vi "Close.vi"(8 "error in (no error)":errorcluster, 11 "HTS221 in":refnum<class "HTS221.lvclass">) -> (0 "error out":errorcluster, 3 "HTS221 out":refnum<class "HTS221.lvclass">)   [LabVIEW 2020, in "HTS221.lvclass"]
doc: "Disables the HTS221"
uses:
  HTS221.lvclass
  LINX I2C/LINX I2C.lvclass
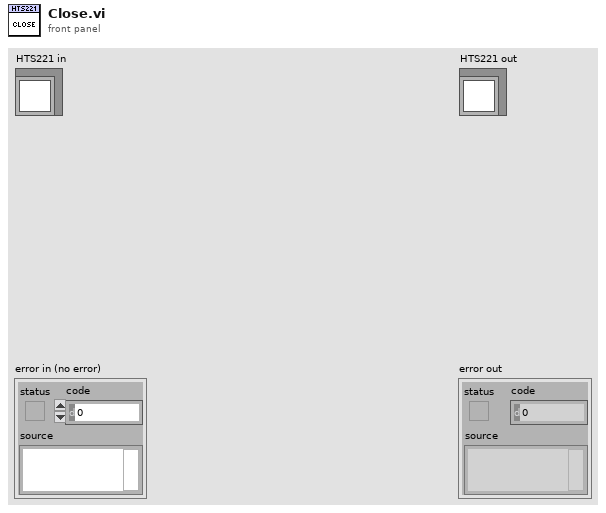
[diagram p1: front panel]
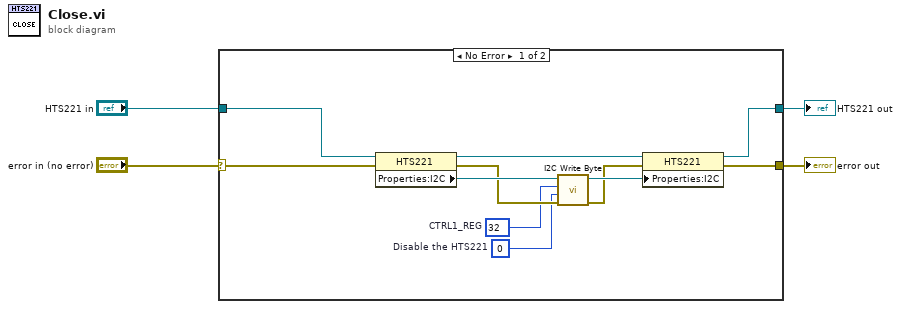
[diagram p0: block diagram]
diagram:
  n1 = case shown="No Error" "error in (no error)" {
    selector: "error in (no error)" -> [w14 w17]
    tunnel: [w7 w17] -> w3
    tunnel: [w6 w16] -> w1
    tunnel: "HTS221 in" -> [w15 w16]
    frame No Error {
      w10 = u8 0  # Disable the HTS221
      w11 = u8 32  # CTRL1_REG
      n2 = property class="HTS221"(reference=w15, error in=w14) -> (reference out=w5:refnum<class "HTS221.lvclass">, error out=w12:errorcluster, "Properties:I2C"=w13:refnum<class "LINX I2C.lvclass">)
      n3 = call "I2C Write Byte.vi"("error in (no error)"=w12, "Value"=w10, "Register Address"=w11, "LINX I2C in"=w13) -> ("error out"=w8:errorcluster, "LINX I2C out"=w9:refnum<class "LINX I2C.lvclass">)  [unwired: 6 in]
      n4 = property class="HTS221"(reference=w5, error in=w8, "Properties:I2C"=w9) -> (reference out=w6:refnum<class "HTS221.lvclass">, error out=w7:errorcluster)
    }
    frame Error {
    }
  }
  "error out" <- w3
  "HTS221 out" <- w1
